vi "Method.vi"(4 "Value":refnum<class "Abs_Value.lvclass">) -> (1 "Result":refnum<class "ConvertTo_Binary.lvclass">)   [LabVIEW 2021, in "ConvertTo_Binary.lvclass"]
uses:
  ConvertTo_Binary.lvclass
  Abs_Types/Value/Abs_Value.lvclass
  ConvertTo_Binary.lvclass/ConvertTo_Binary.ctl
  Properties/Write Value.vi
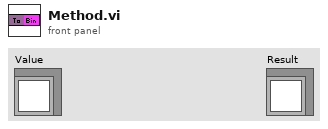
[diagram p1: front panel]
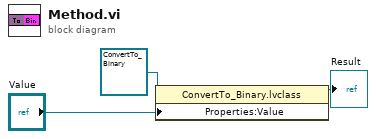
[diagram p0: block diagram]
diagram:
  n1 = property class="ConvertTo_Binary.lvclass"(reference=refnum<class "ConvertTo_Binary.lvclass"> refnum ("ConvertTo_DBL.lvclass"), "Properties:Value"="Value") -> (reference out=→"Result":refnum<class "ConvertTo_Binary.lvclass">)  [unwired: 1 in, 1 out]
